vi "stayOutKeeperArea.vi"(0 "DesireState":T1=enum."FrontWall", 1 "CurrentState":T1=enum."FrontWall", 3 "Dest":dbl[](array[numeric]), 4 "LeftCornerPosition":dbl[](array[numeric]), 5 "error in (no error)":errorcluster, 9 "reference":i32) -> (14 "CorrectDest":dbl[](array[numeric]), 19 "error out":errorcluster)   [LabVIEW 2024, in "DefendAreaTactic.lvclass"]
uses:
  DefendAreaTactic.lvclass
  WallPositions.ctl
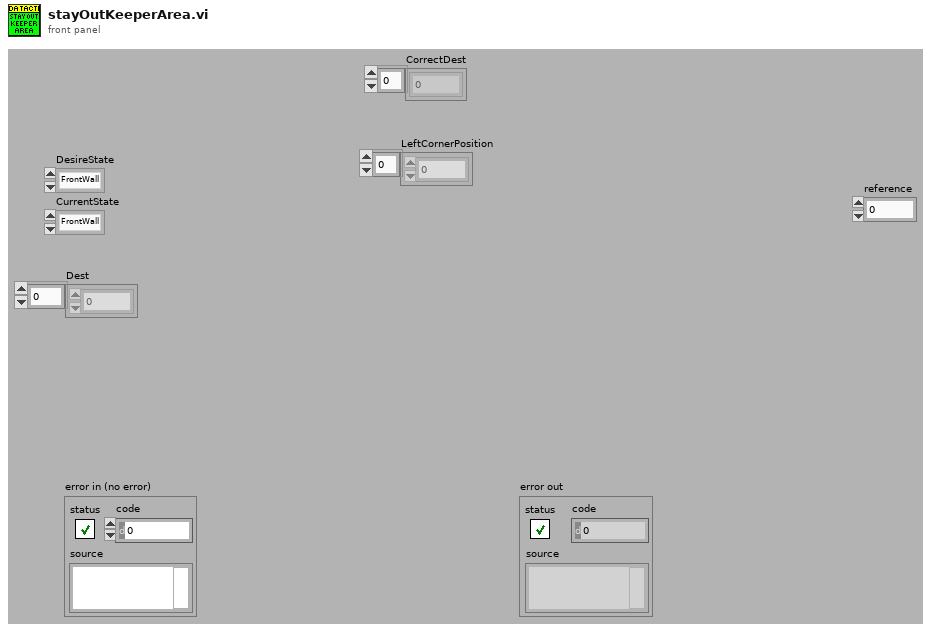
[diagram p1: front panel]
types:
  T1 = typedef "WallPositions.ctl" = enum16{"LeftWall", "LeftCorner", "FrontWall", "RightCorner", "RightWall"}
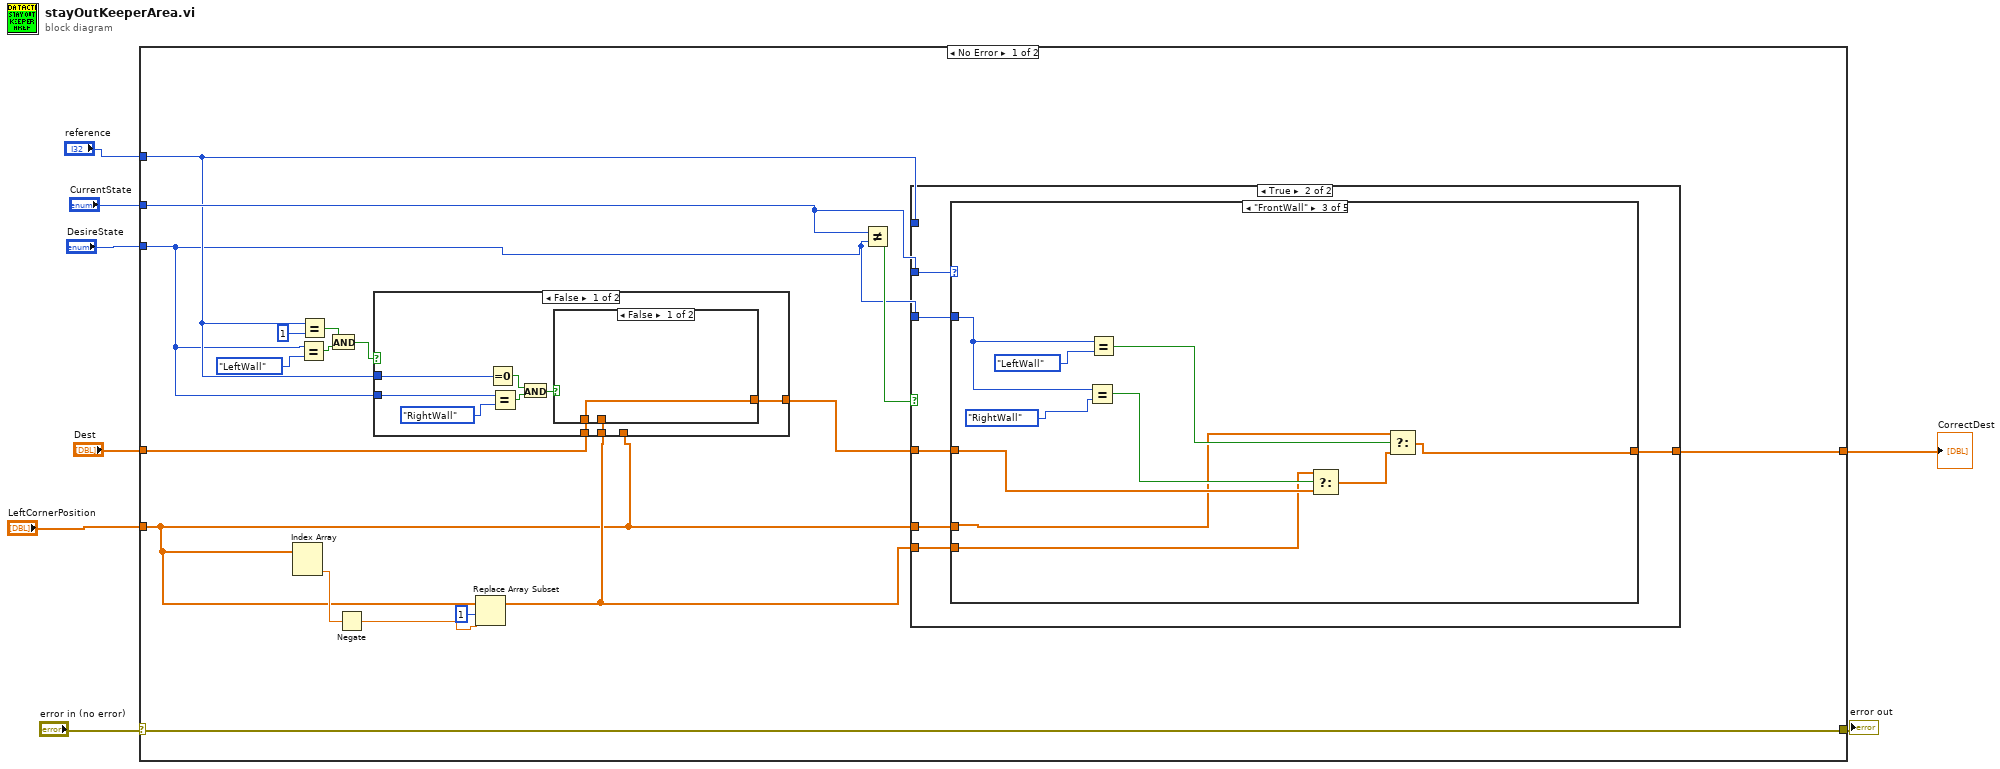
[diagram p0: block diagram]
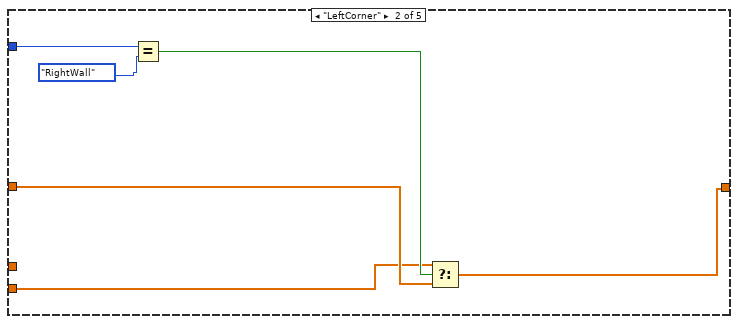
[diagram p6: hidden frame]
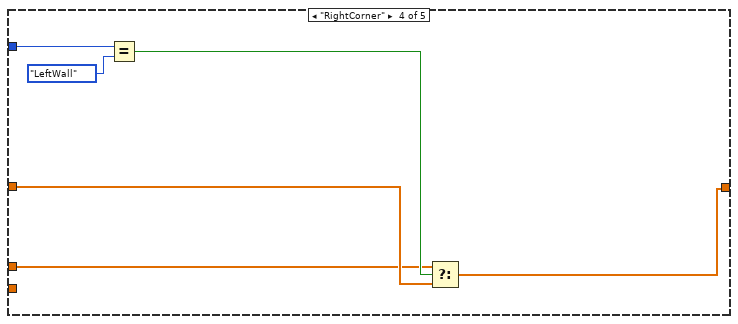
[diagram p7: hidden frame]
diagram:
  n1 = case shown="No Error" "error in (no error)" {
    selector: "error in (no error)" -> [w26 w71]
    tunnel: [w26 w71] -> w7
    tunnel: "DesireState" -> [w11 _]
    tunnel: "CurrentState" -> [w25 _]
    tunnel: "Dest" -> [w19 w70]
    tunnel: [w23 w70] -> w3
    tunnel: "LeftCornerPosition" -> [w9 _]
    tunnel: "reference" -> [w16 _]
    frame No Error {
      n2 = Index Array(array=w9) -> (element #2=w21:dbl)  [unwired: 2 in, 1 out]
      n3 = Equal?(x=w11, y=WallPositions."LeftWall" ("WallState")) -> (x = y?=w17:bool)
      n4 = Equal?(x=w16, y=1) -> (x = y?=w14:bool)
      n5 = And(x=w14, y=w17) -> (x .and. y?=w13:bool)
      n6 = Negate(x=w21) -> (-x=w20:dbl)
      n7 = Replace Array Subset(array=w9, new element=w20, index=1) -> (w10:dbl[])
      n8 = case shown="False" w13 {
        tunnel: w16 -> [w35 _]
        tunnel: w11 -> [w30 _]
        tunnel: w19 -> [w29 _]
        tunnel: [w28 w38] -> w18
        tunnel: w10 -> [w27 _]
        tunnel: w9 -> [_ w38]
        frame False {
          n9 = Equal To 0?(x=w35) -> (x = 0?=w33:bool)
          n10 = Equal?(x=w30, y=WallPositions."RightWall" ("WallState")) -> (x = y?=w32:bool)
          n11 = And(x=w33, y=w32) -> (x .and. y?=w31:bool)
          n12 = case shown="False" w31 {
            tunnel: w29 -> [w36 _]
            tunnel: [w36 w37] -> w28
            tunnel: w27 -> [_ w37]
            frame False {
            }
            frame True {
            }
          }
        }
        frame True {
        }
      }
      n13 = Not Equal?(x=w25, y=w11) -> (x != y?=w24:bool)
      n14 = case shown="True" w24 {
        tunnel: w25 -> [_ w45]
        tunnel: w18 -> [w39 w42]
        tunnel: [w39 w44] -> w23
        tunnel: w9 -> [_ w41]
        tunnel: w11 -> [_ w43]
        tunnel: w10 -> [_ w40]
        tunnel: w16 -> [_ _]
        frame False {
        }
        frame True {
          n15 = case shown="\"FrontWall\"" w45 {
            tunnel: [w46 w51 w56 w67 w69] -> w44
            tunnel: w43 -> [_ w50 w61 w66 _]
            tunnel: w42 -> [_ w52 w57 w68 _]
            tunnel: w41 -> [w46 _ w53 w63 _]
            tunnel: w40 -> [_ w47 w54 _ w69]
            frame "LeftWall", Default {
            }
            frame "LeftCorner" {
              n16 = Equal?(x=w50, y=WallPositions."RightWall" ("WallState")) -> (x = y?=w49:bool)
              n17 = Select(t=w47, s=w49, f=w52) -> (s? t:f=w51:dbl[])
            }
            frame "FrontWall" {
              n18 = Equal?(x=w61, y=WallPositions."RightWall" ("WallState")) -> (x = y?=w59:bool)
              n19 = Equal?(x=w61, y=WallPositions."LeftWall" ("WallState")) -> (x = y?=w60:bool)
              n20 = Select(t=w54, s=w59, f=w57) -> (s? t:f=w58:dbl[])
              n21 = Select(t=w53, s=w60, f=w58) -> (s? t:f=w56:dbl[])
            }
            frame "RightCorner" {
              n22 = Equal?(x=w66, y=WallPositions."LeftWall" ("WallState")) -> (x = y?=w65:bool)
              n23 = Select(t=w63, s=w65, f=w68) -> (s? t:f=w67:dbl[])
            }
            frame "RightWall" {
            }
          }
        }
      }
    }
    frame Error {
    }
  }
  "error out" <- w7
  "CorrectDest" <- w3
